vi "E02_EstructuraWhile.vi"() -> ()   [LabVIEW 2026]
panel:
  in  "stop":bool
  out "Waveform Chart":dbl(graph)
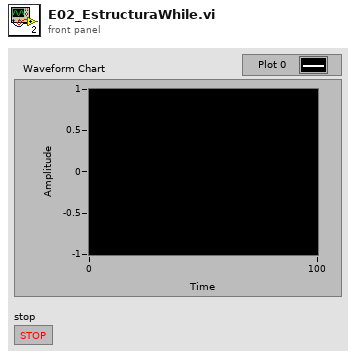
[diagram p1: front panel]
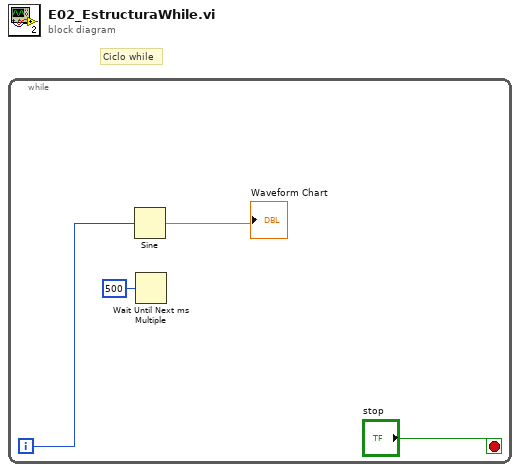
[diagram p0: block diagram]
diagram:
  # "Ciclo while"
  n1 = while {
    i -> [w3]
    stop <- "stop" stop-if-true
    n2 = Sine(x=w3) -> (sin(x)=→"Waveform Chart":dbl)
    n3 = Wait Until Next ms Multiple(millisecond multiple=u32 500) -> ()  [unwired: 1 out]
  }
